vi "OpenRingFiles.vi"(2 "Ring Number":i32, 3 "Save Options":T2={"Save h Files?"=FALSE, "Used Saved h?"=FALSE, "Save image data?"=FALSE, "Path"=path "F:/Test"}, 4 "Variables":T1={"Number of rings"=1, "sound spd (cm/s)"=150000, "z span (cm)"=4.0, "z steps"=20, "y spacing (cm)"=0.01, "y steps"=50, "time step (s)"=1e-08, "z"=0.0, "y"=0.0, "ref delay"=0.0, "freq (MHz)"=4.71, "cycles"=300} {"freq (MHz)" format="%.2f"; "z span (cm)" format="%.2f"; "y" format="%.2f"; "ref delay" format="%.2f"; "y spacing (cm)" format="%.3f"; "z" format="%.2f"; "time step (s)" format="%.2e"}) -> (0 "Y axis":dbl[](array[numeric]) format="%.2f", 1 "h(r,t)":dbl[][](array[numeric]) format="%.2f")   [LabVIEW 2022 SP3]
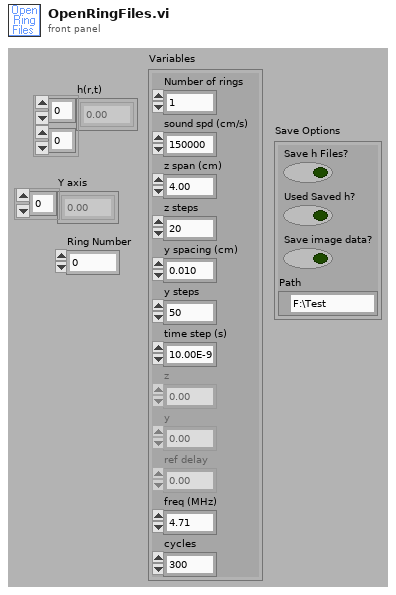
[diagram p1: front panel]
types:
  T1 = cluster{"Number of rings":i32, "sound spd (cm/s)":i32, "z span (cm)":dbl, "z steps":i32, "y spacing (cm)":dbl, "y steps":i32, "time step (s)":sgl, "z":dbl, "y":dbl, "ref delay":dbl, "freq (MHz)":dbl, "cycles":i32}
  T2 = cluster{"Save h Files?":bool, "Used Saved h?":bool, "Save image data?":bool, "Path":path}
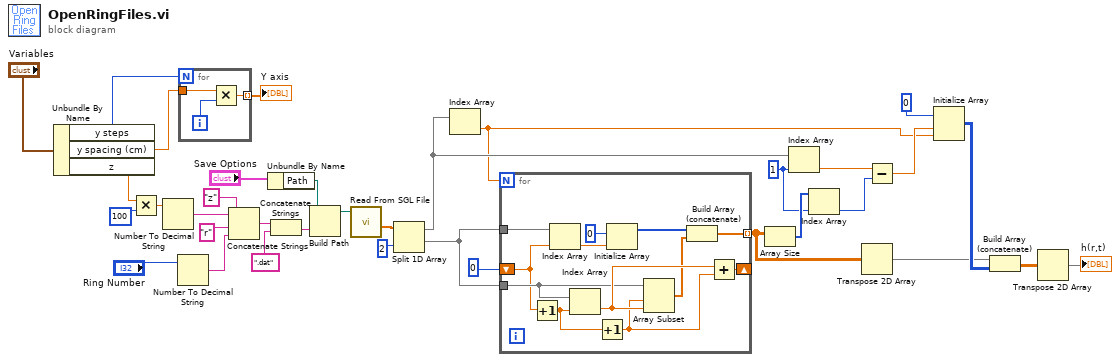
[diagram p0: block diagram]
diagram:
  w21 = 1
  n1 = Unbundle By Name("Variables") -> ("y steps"=w7:i32, "y spacing (cm)"=w8:dbl, "z"=w35:dbl)
  n2 = Multiply(x=w35, y=100) -> (x*y=w33:dbl)
  n3 = Number To Decimal String(number=w33) -> (decimal integer string=w32:string)  [unwired: 1 out]
  n4 = Number To Decimal String(number="Ring Number") -> (decimal integer string=w29:string)  [unwired: 1 out]
  n5 = for {
    N: w7 -> [_]
    tunnel: [w36] -> w6 mode=indexing
    tunnel: w8 -> [w37]
    i -> [w38]
    n6 = Multiply(x=w37, y=w38) -> (x*y=w36:dbl)
  }
  "Y axis" <- w6
  n7 = Concatenate Strings("z", w32, "r", w29) -> (w27:string)
  n8 = Unbundle By Name("Save Options") -> ("Path"=w4:path)
  n9 = Concatenate Strings(w27, ".dat") -> (w25:string)
  n10 = Build Path(base path=w4, name or relative path=w25) -> (appended path=w2:path)
  n11 = call <vilib>:"Read From SGL File.vi"("file path (dialog if empty)"=w2) -> ("1D array"=w1:sgl[])  [unwired: 2 in, 8 out]
  n12 = Split 1D Array(array=w1, index=2) -> (first subarray=w16:sgl[], second subarray=w10:sgl[])
  n13 = Index Array(array=w16) -> (element=w11:sgl)  [unwired: 1 in]
  n14 = for {
    N: w11 -> [_]
    tunnel: w10 -> [w44]
    shift-right: [w47] -> _
    shift-left: 0 -> [w41]
    tunnel: [w42] -> w15 mode=indexing
    tunnel: w10 -> [w43]
    n15 = Increment(x=w41) -> (x+1=w40:sgl)
    n16 = Index Array(array=w44, index=w41) -> (element=w49:sgl)
    n17 = Index Array(array=w43, index=w40) -> (element=w48:sgl)
    n18 = Increment(x=w40) -> (x+1=w39:sgl)
    n19 = Initialize Array(0, w49) -> (w46:i32[])
    n20 = Array Subset(array=w43, index=w39, length=w48) -> (w45:sgl[])
    n21 = Build Array (concatenate)(w46, w45) -> (w42:sgl[])
    n22 = Add(x=w48, y=w39) -> (x+y=w47:sgl)
  }
  n23 = Array Size(array=w15) -> (size(s)=w22:i32[])
  n24 = Index Array(array=w16, index=w21) -> (element=w20:sgl)
  n25 = Index Array(array=w22, index=w21) -> (element=w19:i32)
  n26 = Transpose 2D Array(2D array=w15) -> (transposed array=w13:sgl[][])
  n27 = Subtract(x=w20, y=w19) -> (x-y=w12:sgl)
  n28 = Initialize Array(0, w12, w11) -> (w17:i32[][])
  n29 = Build Array (concatenate)(w13, w17) -> (w14:sgl[][])
  n30 = Transpose 2D Array(2D array=w14) -> (transposed array=→"h(r,t)":sgl[][])
